vi "Expand Section Range.vi"(3 "Section Range":string) -> (0 "Section IDs":i32[](array[numeric]), 1 "Section End Points":i32[](array[numeric]))   [LabVIEW 2020, in "AoC 2022.lvlib"]
doc: "<B>Input</B>\n<B>Section Range</B>: 2-8\n\n<B>Output</B>\n<B>Section End Points</B>: [2, 8]\n<B>Section IDs</B>: [2, 3, 4, 5, 6, 7, 8]"
uses:
  AoC 2022.lvlib
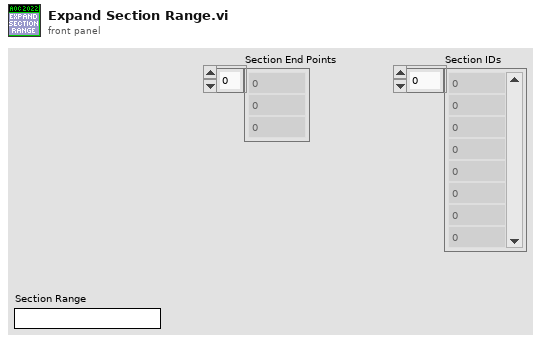
[diagram p1: front panel]
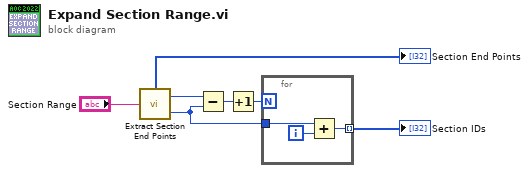
[diagram p0: block diagram]
diagram:
  n1 = call "Extract Section End Points.vi"("Section Range"="Section Range") -> ("Section End Points"=→"Section End Points":i32[], "Section End"=w2:i32, "Section Start"=w3:i32)
  n2 = Subtract(x=w2, y=w3) -> (x-y=w7:i32)
  n3 = Increment(x=w7) -> (x+1=w5:i32)
  n4 = for {
    N: w5 -> [_]
    tunnel: w3 -> [w10]
    tunnel: [w8] -> w6 mode=indexing
    i -> [w9]
    n5 = Add(x=w10, y=w9) -> (x+y=w8:i32)
  }
  "Section IDs" <- w6
